vi "题目1.vi"() -> ()   [LabVIEW 2017]
panel:
  out "元素 4":dbl
  out "元素 3":dbl
  out "元素 2":dbl
  out "元素":dbl
  out "添加的数组":dbl[](array[numeric])
  out "数组":dbl[](array[numeric])
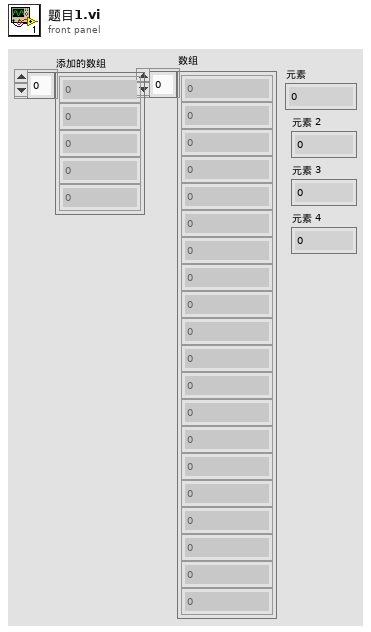
[diagram p1: front panel]
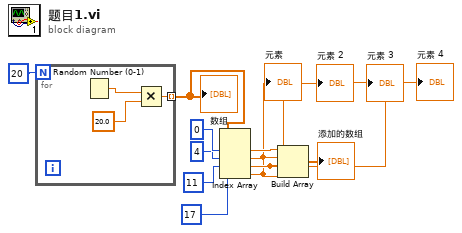
[diagram p0: block diagram]
diagram:
  n1 = for {
    N: 20 -> [_]
    tunnel: [w12] -> w6 mode=indexing
    n2 = Random Number (0-1)() -> (number: 0 to 1=w13:dbl)
    n3 = Multiply(x=w13, y=20.0) -> (x*y=w12:dbl)
  }
  "数组" <- w6
  n4 = Index Array(array=w6, index #1=0 ("索引"), index #2=4 ("索引"), index #3=11 ("索引"), index #4=17 ("索引")) -> (element #1=w5:dbl, element #2=w4:dbl, element #3=w3:dbl, element #4=w2:dbl)
  "元素" <- w5
  "元素 2" <- w4
  "元素 3" <- w3
  "元素 4" <- w2
  n5 = Build Array(w5, w4, w3, w2) -> (→"添加的数组":dbl[])
